vi "VG_SN.vi"() -> ()   [LabVIEW 2020]
panel:
  out "VG SN":string
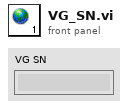
[diagram p1: front panel]
diagram:
